vi "Dispatch_FindOrFilterOnName.vi"(9 "vi path":path, 10 "Data Tree":refnum<vi>, 11 "SubPanel in":refnum<vi>) -> (0 "error out":errorcluster)   [LabVIEW 2013, in "FindName Task_Manager.lvlib"]
uses:
  FindName Task_Manager.lvlib
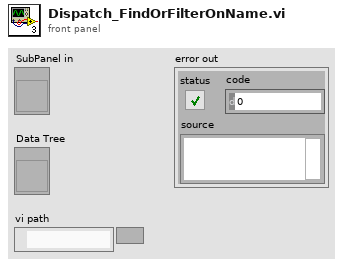
[diagram p1: front panel]
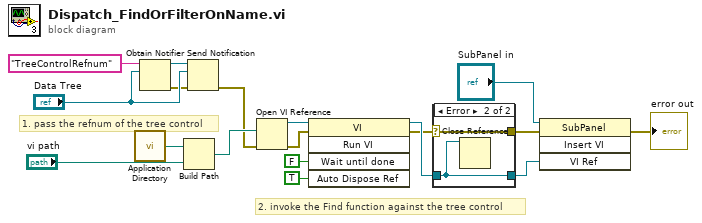
[diagram p0: block diagram]
diagram:
  # "2. invoke the Find function against the tree control"
  # "1. pass the refnum of the tree control"
  n1 = call <vilib>:"Application Directory.vi"() -> ("Application Directory"=w13:path)
  n2 = Obtain Notifier(name (unnamed)="TreeControlRefnum", notification data type="Data Tree") -> (notifier out=w2:refnum<notifier>, error out=w3:errorcluster)  [unwired: 2 in, 1 out]
  n3 = Build Path(base path=w13, name or relative path="vi path") -> (appended path=w12:path)
  n4 = Send Notification(notification="Data Tree", notifier=w2, error in (no error)=w3) -> (error out=w5:errorcluster)  [unwired: 1 out]
  n5 = Open VI Reference(vi path=w12, error in (no error)=w5) -> (vi reference=w7:refnum<vi>, error out=w9:errorcluster)  [unwired: 4 in]
  n6 = invoke class="VI" method="Run VI"(reference=w7, error in=w9, "Wait until done"=FALSE ("Wait Until Done"), "Auto Dispose Ref"=TRUE ("Auto Dispose Reference")) -> (reference out=w15:refnum<vi>, error out=w14:errorcluster)  [unwired: 1 in, 3 out]
  n7 = case shown="Error" w14 {
    selector: w14 -> [w20 w22]
    tunnel: [w20 w22] -> w17
    tunnel: w15 -> [w19 w21]
    tunnel: [w19 w21] -> w16
    frame No Error {
    }
    frame Error {
      n8 = Close Reference(reference=w21) -> ()  [unwired: 1 in, 1 out]
    }
  }
  n9 = invoke on="Invoke Node" class="SubPanel" method="Insert VI"(reference="SubPanel in", error in=w17, "VI Ref"=w16) -> (error out=→"error out":errorcluster)  [unwired: 1 in, 3 out]
